vi "startHW.vi"(8 "error in (no error)":errorcluster, 11 "Model in":refnum<class "Model.lvclass">) -> (0 "error out":errorcluster, 3 "Model out":refnum<class "Model.lvclass">)   [LabVIEW 2016, in "Model.lvclass"]
doc: "On first call, starts the hardware .\n\nFor a real-time application,the FPGA VI reference is unique to each component."
uses:
  Model.lvclass
  Model.lvclass/Model.ctl
  Target/Target/Target.lvclass
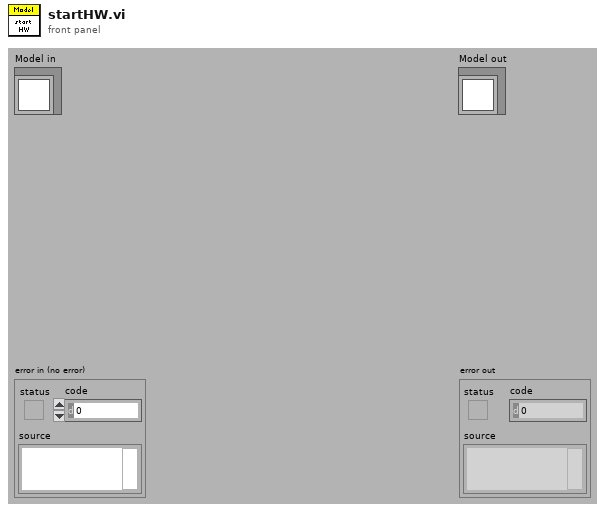
[diagram p1: front panel]
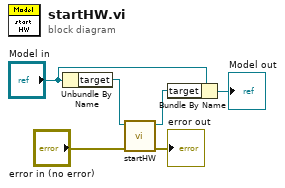
[diagram p0: block diagram]
diagram:
  n1 = Unbundle By Name("Model in") -> ("target"=w6:refnum<class "Target.lvclass">)
  n2 = call-dynamic "startHW.vi"("error in (no error)"="error in (no error)", "Target in"=w6) -> ("error out"=→"error out":errorcluster, "Target out"=w3:refnum<class "Target.lvclass">)  [unwired: 8 in]
  n3 = Bundle By Name(cluster="Model in", "target"=w3) -> (→"Model out":refnum<class "Model.lvclass">)
